vi "Decimate Plot Array.vi"(4 "Y Dimension":i32, 6 "X Dimension":i32, 10 "Color Index Array In":i32[](array[numeric]), 11 "Vertex Array In":cluster{"X":sgl, "Y":sgl, "Z":sgl}[](array[cluster])) -> (2 "Color Index Array Out":i32[](array[numeric]), 3 "Vertex Array Out":cluster{"X":sgl, "Y":sgl, "Z":sgl}[](array[cluster]))   [LabVIEW 2017, in "3D Plot.lvclass"]
uses:
  <vilib>/Math Plots/3D Math Plots/3D Plot/3D Plot/3D Plot.lvclass
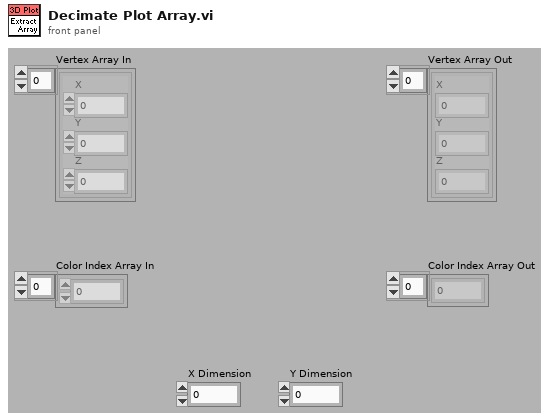
[diagram p1: front panel]
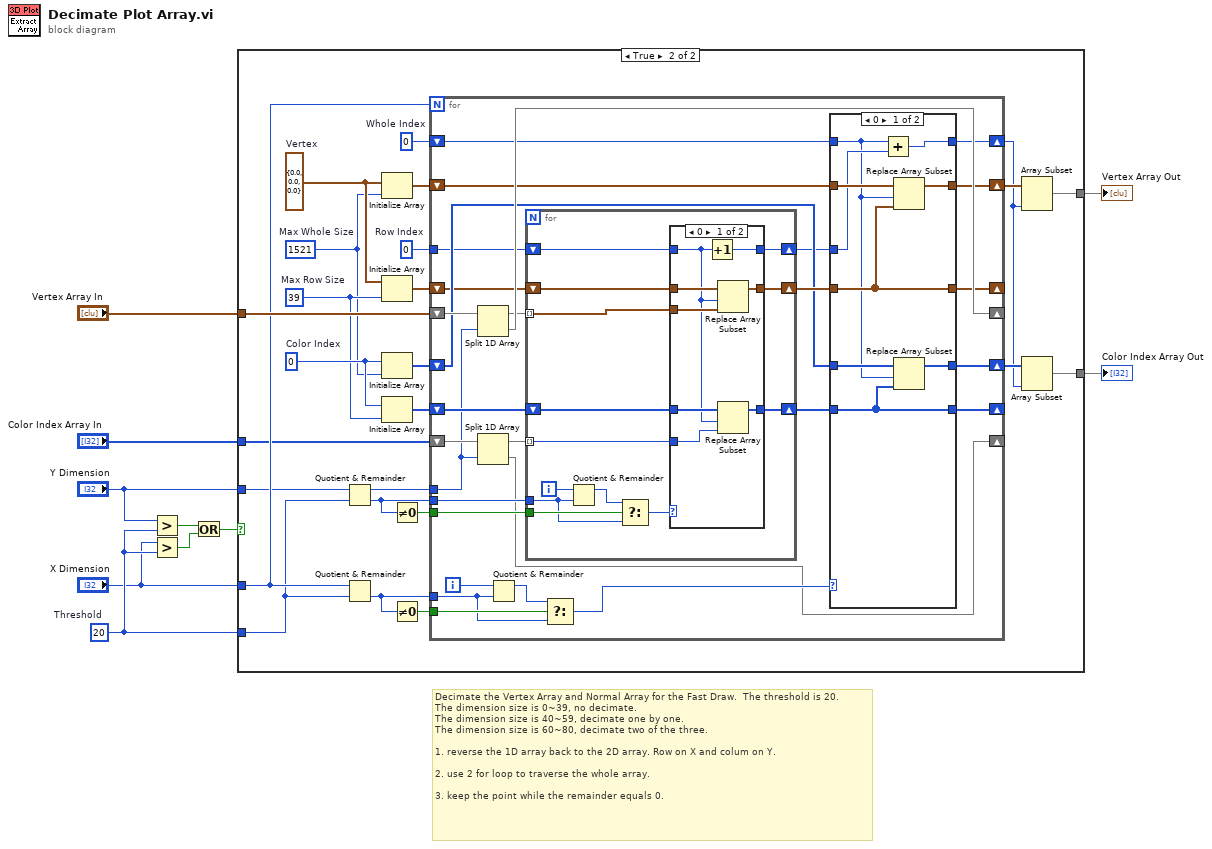
[diagram p0: block diagram]
diagram:
  w7 = 20  # Threshold
  # "Decimate the Vertex Array and Normal Array for the Fast Draw.  The threshold is 20.\nThe dimension size is 0~39, no decimate.\nThe dimension size is 40~59, decimate one by one.\nThe dimension size is 60~80, decimate two of the three.\n\n1. reverse the 1D array back to the 2D array. Row on X and colum on Y.\n\n2. use 2 for loop to traverse the whole array. \n\n3. keep the point while the remainder equals 0."
  n1 = Greater?(x="Y Dimension", y=w7) -> (0:w4:bool)
  n2 = Greater?(x="X Dimension", y=w7) -> (0:w3:bool)
  n3 = Or(x=w4, y=w3) -> (x .or. y?=w5:bool)
  n4 = case shown="True" w5 {
    tunnel: "Vertex Array In" -> [w12 w36]
    tunnel: "X Dimension" -> [_ w35]
    tunnel: "Y Dimension" -> [_ w34]
    tunnel: [w12 w14] -> w9
    tunnel: w7 -> [_ w28]
    tunnel: "Color Index Array In" -> [w11 w27]
    tunnel: [w11 w13] -> w1
    frame False {
    }
    frame True {
      w16 = 1521  # Max Whole Size
      w18 = 0  # Whole Index
      w19 = 0  # Row Index
      w20 = 39  # Max Row Size
      w21 = cluster{"X":sgl, "Y":sgl, "Z":sgl} {"X"=0.0, "Y"=0.0, "Z"=0.0}  # Vertex
      w23 = 0  # Color Index
      n5 = Quotient & Remainder(x=w34, y=w28) -> (floor(x/y)=w29:i32)  [unwired: 1 out]
      n6 = Quotient & Remainder(x=w35, y=w28) -> (floor(x/y)=w32:i32)  [unwired: 1 out]
      n7 = Initialize Array(w21, w16) -> (w26:cluster{"X":sgl, "Y":sgl, "Z":sgl}[])
      n8 = Initialize Array(w21, w20) -> (w24:cluster{"X":sgl, "Y":sgl, "Z":sgl}[])
      n9 = Initialize Array(w23, w16) -> (w25:i32[])
      n10 = Initialize Array(w23, w20) -> (w22:i32[])
      n11 = Not Equal To 0?(x=w29) -> (x != 0?=w30:bool)
      n12 = Not Equal To 0?(x=w32) -> (x != 0?=w31:bool)
      n13 = for {
        N: w35 -> [_]
        shift-right: [w63] -> _
        shift-left: w36 -> [w64]
        shift-right: [w61] -> w33
        shift-left: w26 -> [w62]
        tunnel: w34 -> [w37]
        tunnel: w29 -> [w58]
        tunnel: w32 -> [w55]
        tunnel: w31 -> [w56]
        tunnel: w30 -> [w52]
        shift-right: [w48] -> _
        shift-left: w27 -> [w49]
        shift-right: [w46] -> w17
        shift-left: w25 -> [w47]
        shift-right: [w43] -> _
        shift-left: w24 -> [w45]
        shift-right: [w42] -> _
        shift-left: w22 -> [w44]
        tunnel: w19 -> [w41]
        shift-right: [w39] -> w15
        shift-left: w18 -> [w40]
        i -> [w60]
        n14 = Split 1D Array(array=w64, index=w37) -> (first subarray=w59:cluster{"X":sgl, "Y":sgl, "Z":sgl}[], second subarray=w63:cluster{"X":sgl, "Y":sgl, "Z":sgl}[])
        n15 = Split 1D Array(array=w49, index=w37) -> (first subarray=w50:i32[], second subarray=w48:i32[])
        n16 = Quotient & Remainder(x=w60, y=w55) -> (x-y*floor(x/y)=w54:i32)  [unwired: 1 out]
        n17 = for {
          tunnel: w59 -> [w76] mode=indexing
          tunnel: w58 -> [w70]
          shift-right: [w75] -> w57
          shift-left: w45 -> [w74]
          tunnel: w52 -> [w73]
          tunnel: w50 -> [w67] mode=indexing
          shift-right: [w68] -> w51
          shift-left: w44 -> [w69]
          shift-right: [w65] -> w38
          shift-left: w41 -> [w66]
          i -> [w77]
          n18 = Quotient & Remainder(x=w77, y=w70) -> (x-y*floor(x/y)=w72:i32)  [unwired: 1 out]
          n19 = Select(t=w72, s=w73, f=w70) -> (s? t:f=w71:i32)
          n20 = case shown="0" w71 {
            tunnel: w74 -> [w85 w88]
            tunnel: w76 -> [w80 _]
            tunnel: [w84 w88] -> w75
            tunnel: w69 -> [w82 w87]
            tunnel: w67 -> [w81 _]
            tunnel: [w83 w87] -> w68
            tunnel: w66 -> [w78 w86]
            tunnel: [w79 w86] -> w65
            frame 0 {
              n21 = Increment(x=w78) -> (x+1=w79:i32)
              n22 = Replace Array Subset(array=w85, new element=w80, index=w78) -> (w84:cluster{"X":sgl, "Y":sgl, "Z":sgl}[])
              n23 = Replace Array Subset(array=w82, new element=w81, index=w78) -> (w83:i32[])
            }
            frame 1, Default {
            }
          }
        }
        n24 = Select(t=w54, s=w56, f=w55) -> (s? t:f=w53:i32)
        n25 = case shown="0" w53 {
          tunnel: w62 -> [w97 w102]
          tunnel: [w96 w102] -> w61
          tunnel: w57 -> [w93 w99]
          tunnel: w51 -> [w92 w100]
          tunnel: [w95 w101] -> w46
          tunnel: w47 -> [w94 w101]
          tunnel: [w93 w99] -> w43
          tunnel: [w92 w100] -> w42
          tunnel: w40 -> [w89 w98]
          tunnel: [w91 w98] -> w39
          tunnel: w38 -> [w90 _]
          frame 0 {
            n26 = Add(x=w89, y=w90) -> (x+y=w91:i32)
            n27 = Replace Array Subset(array=w97, new element=w93, index=w89) -> (w96:cluster{"X":sgl, "Y":sgl, "Z":sgl}[])
            n28 = Replace Array Subset(array=w94, new element=w92, index=w89) -> (w95:i32[])
          }
          frame 1, Default {
          }
        }
      }
      n29 = Array Subset(array=w33, length=w15) -> (w14:cluster{"X":sgl, "Y":sgl, "Z":sgl}[])  [unwired: 1 in]
      n30 = Array Subset(array=w17, length=w15) -> (w13:i32[])  [unwired: 1 in]
    }
  }
  "Vertex Array Out" <- w9
  "Color Index Array Out" <- w1
